vi "SHA-2-U32.vi"(7 "Type":T1, 8 "error in (no error)":errorcluster, 11 "Message":u8[](array[numeric])) -> (0 "error out":errorcluster, 1 "ASCII formatted hash":string, 3 "Hash":u8[](array[numeric]))   [LabVIEW 2011, in "i3-external-encryption.lvlib"]
doc: "Performs a SHA-2 U32 hash action.\n\n(c) Ton Plomp, 2011\nTHIS SOFTWARE IS PROVIDED AS IS, AND ANY WARRANTY IS REJECTED"
uses:
  i3-external-encryption.lvlib
  SHA-2_U32_types.ctl
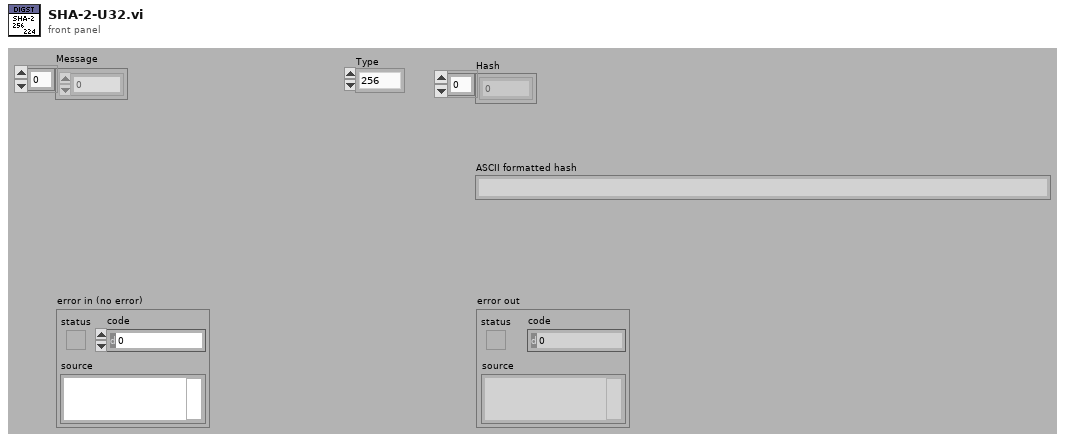
[diagram p1: front panel]
types:
  T1 = typedef "i3-external-encryption.lvlib/SHA-2_U32_types.ctl" = enum16{"256", "224"}
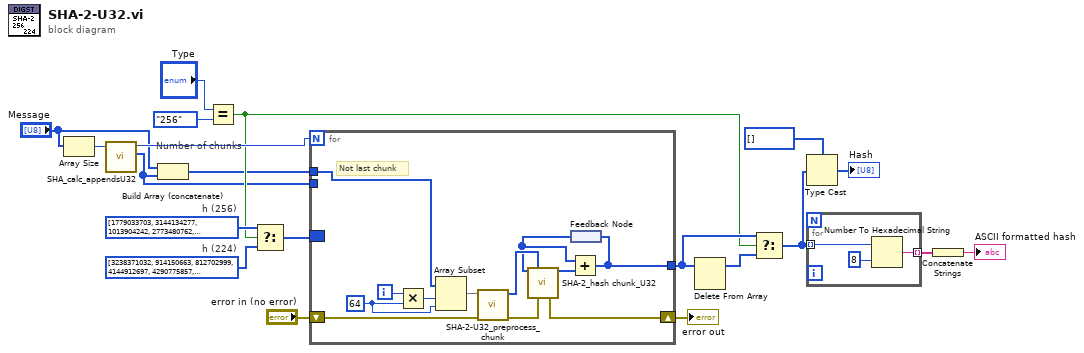
[diagram p0: block diagram]
diagram:
  w10 = u32[] [3238371032, 914150663, 812702999, 4144912697, 4290775857, 1750603025, 1694076839, 3204075428]  # h (224)
  w12 = u32[] [1779033703, 3144134277, 1013904242, 2773480762, 1359893119, 2600822924, 528734635, 1541459225]  # h (256)
  # "Number of chunks"
  n1 = Array Size(array="Message") -> (size(s)=w19:i32)
  n2 = call "SHA_calc_appendsU32.vi"("String length"=w19) -> ("Append"=w6:u8[], "Number of chunks"=w20:i32)  [unwired: 9 in]
  n3 = Build Array (concatenate)("Message", w6) -> (w4:u8[])
  n4 = Equal?(x="Type", y=SHA-2_U32_types."256" ("Type")) -> (x = y?=w7:bool)
  n5 = Select(t=w12, s=w7, f=w10) -> (s? t:f=w11:u32[])
  n6 = for {
    N: w20 -> [_]
    tunnel: w4 -> [w32]
    tunnel: w6 -> [_]
    tunnel: [w22] -> w9
    border: w11 -> [_]
    shift-right: [w26] -> w18
    shift-left: "error in (no error)" -> [w25]
    i -> [w29]
    w30 = 64 ("x")
    # "Not last chunk"
    n7 = Multiply(x=w29, y=w30) -> (x*y=w31:i32)
    n8 = Array Subset(array=w32, index=w31, length=w30) -> (w27:u8[])
    n9 = call "SHA-2-U32_preprocess_chunk.vi"("error in (no error)"=w25, "Chunk in"=w27) -> ("error out"=w23:errorcluster, "Processed chunk out"=w24:u32[])  [unwired: 8 in]
    n10 = feedback #1() -> (w21:u32[])
    n11 = call "SHA-2_hash chunk_U32.vi"("h in"=w21, "Chunk"=w24, "error in (no error)"=w23) -> ("h out"=w28:u32[], "error out"=w26:errorcluster)  [unwired: 11 in]
    n12 = Add(x=w21, y=w28) -> (x+y=w22:u32[])
    n13 = feedback-in #1(w22) -> ()
  }
  "error out" <- w18
  n14 = Delete From Array(array=w9) -> (array with subset deleted=w8:u32[])  [unwired: 2 in, 1 out]
  n15 = Select(t=w9, s=w7, f=w8) -> (s? t:f=w3:u32[])
  n16 = Type Cast(type=u8[] [] ("binary string hash"), x=w3) -> (*(type *) &x=→"Hash":u8[])
  n17 = for {
    tunnel: w3 -> [w35] mode=indexing
    tunnel: [w33] -> w16 mode=indexing
    n18 = Number To Hexadecimal String(1:i16 8 ("width (-)"), 2:w35) -> (0:w33:string)
  }
  n19 = Concatenate Strings(w16) -> (→"ASCII formatted hash":string)
